vi "GenerateECGvector_V2.vi"(8 "Position_ECG_vector":i32, 9 "ECG_vector":dbl[](array[numeric]), 10 "cooldown In":i64, 11 "EXG1-EXG2 current block":dbl[](array[numeric])) -> (0 "Position_ECG_vector_OUT":i32, 1 "ECG_vector_OUT":dbl[](array[numeric]), 2 "cooldown out":i64)   [LabVIEW 2022 SP3]
panel:
  # "Input"
  # "output"
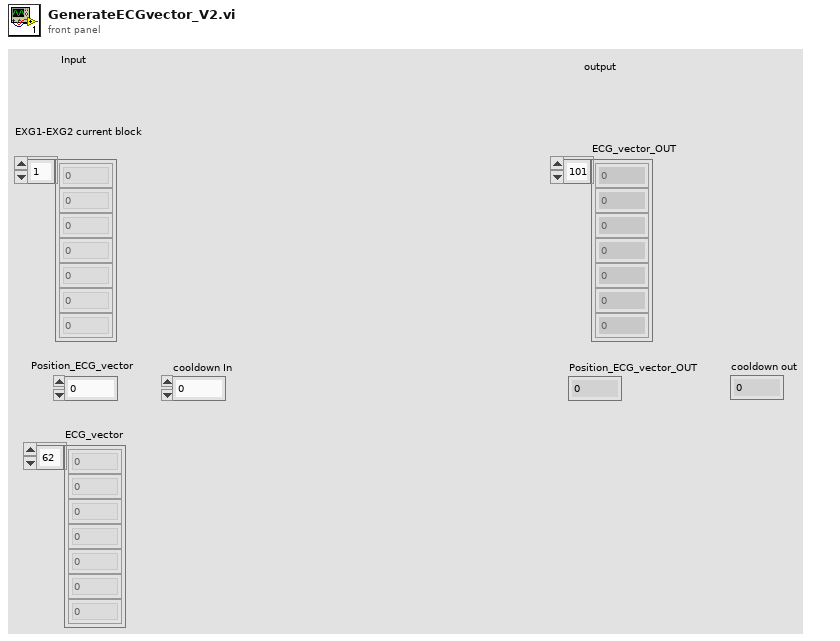
[diagram p1: front panel]
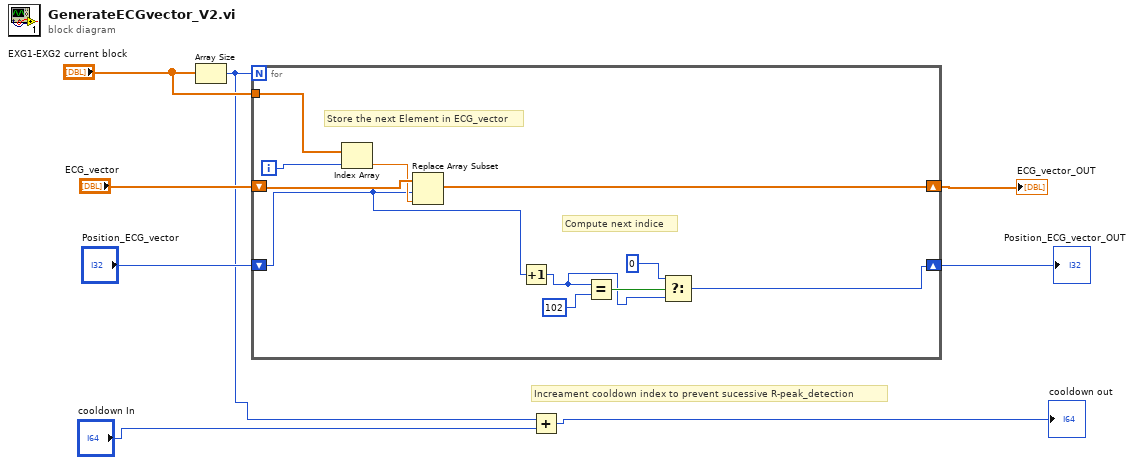
[diagram p0: block diagram]
diagram:
  # "Increament cooldown index to prevent sucessive R-peak_detection"
  n1 = Array Size(array="EXG1-EXG2 current block") -> (size(s)=w1:i32)
  n2 = for {
    N: w1 -> [_]
    shift-right: [w9] -> w4
    shift-left: "Position_ECG_vector" -> [w14]
    shift-right: [w16] -> w5
    shift-left: "ECG_vector" -> [w19]
    tunnel: "EXG1-EXG2 current block" -> [w18]
    i -> [w15]
    # "Compute next indice"
    # "Store the next Element in ECG_vector"
    n3 = Index Array(array=w18, index=w15) -> (element=w17:dbl)
    n4 = Replace Array Subset(array=w19, new element=w17, index=w14) -> (w16:dbl[])
    n5 = Increment(x=w14) -> (x+1=w10:i32)
    n6 = Equal?(x=w10, y=102) -> (x = y?=w12:bool)
    n7 = Select(t=0, s=w12, f=w10) -> (s? t:f=w9:i32)
  }
  "ECG_vector_OUT" <- w5
  "Position_ECG_vector_OUT" <- w4
  n8 = Add(x=w1, y="cooldown In") -> (x+y=→"cooldown out":i64)
